vi "Get All VIs in Memory.vi"(8 "错误输入（无错误）":errorcluster, 11 "应用程序引用":refnum<vi>) -> (0 "错误输出":errorcluster, 1 "导出的VI":string[](array[string]), 2 "所有内存中的VI":string[](array[string]), 3 "引用输出":refnum<vi>)   [LabVIEW 2012, in "Application.lvlib"]
uses:
  Application.lvlib
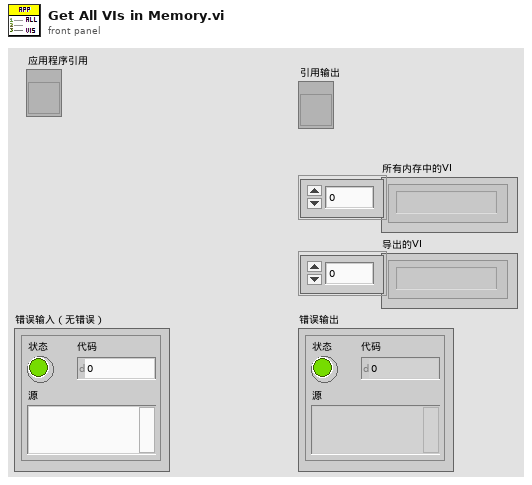
[diagram p1: front panel]
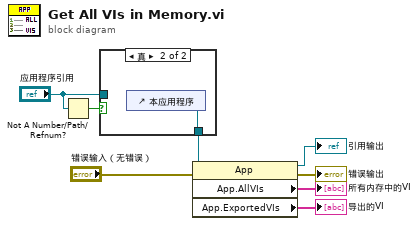
[diagram p0: block diagram]
diagram:
  n1 = Not A Number/Path/Refnum?(number/path/refnum="应用程序引用") -> (NaN/Path/Refnum?=w4:bool)
  n2 = case shown="真" w4 {
    tunnel: "应用程序引用" -> [w9 _]
    tunnel: [w9 w10] -> w2
    frame False {
    }
    frame True {
      n3 = control-ref of="本应用程序"() -> (w10:refnum<vi>)
    }
  }
  n4 = property class="App"(reference=w2, error in="错误输入（无错误）") -> (reference out=→"引用输出":refnum<vi>, error out=→"错误输出":errorcluster, "App.AllVIs"=→"所有内存中的VI":string[], "App.ExportedVIs"=→"导出的VI":string[])
